vi "comm control flags.vi"(1 "control flags cluster":T1) -> (0 "Control Flags":u32 format="%.0x")   [LabVIEW 2009, in "lvserial.lvlib"]
uses:
  lvserial.lvlib
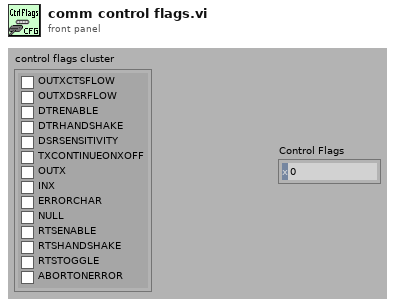
[diagram p1: front panel]
types:
  T1 = cluster{"OUTXCTSFLOW":bool, "OUTXDSRFLOW":bool, "DTRENABLE":bool, "DTRHANDSHAKE":bool, "DSRSENSITIVITY":bool, "TXCONTINUEONXOFF":bool, "OUTX":bool, "INX":bool, "ERRORCHAR":bool, "NULL":bool, "RTSENABLE":bool, "RTSHANDSHAKE":bool, "RTSTOGGLE":bool, "ABORTONERROR":bool}
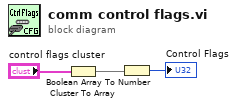
[diagram p0: block diagram]
diagram:
  n1 = Cluster To Array(cluster="control flags cluster") -> (array=w1:bool[])
  n2 = Boolean Array To Number(Boolean array=w1) -> (number=→"Control Flags":u32)
